vi "Write Pressure Alarm Level.vi"(8 "error in (no error)":errorcluster, 10 "Pressure Alarm Level":dbl format="%^_3g", 11 "Pressure Monitor in":refnum<class "Pressure Monitor.lvclass">) -> (0 "error out":errorcluster, 3 "Pressure Monitor out":refnum<class "Pressure Monitor.lvclass">)   [LabVIEW 2022 SP3, in "Pressure Monitor.lvclass"]
uses:
  Pressure Monitor.lvclass
  Pressure Monitor.lvclass/Pressure Monitor.ctl
  Pressure Settings.ctl
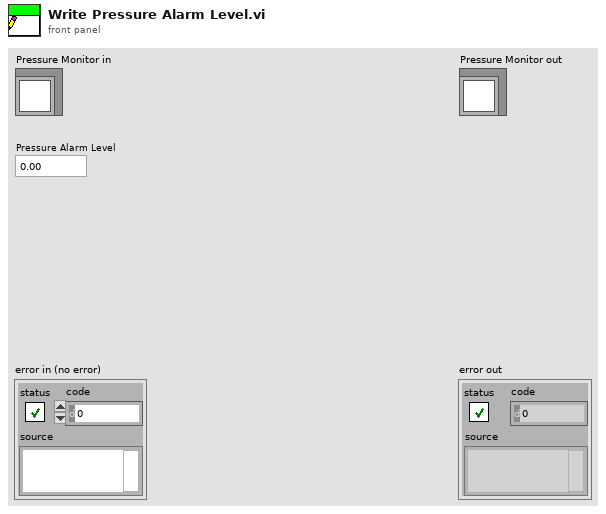
[diagram p1: front panel]
types:
  T1 = typedef "Pressure Monitor.lvclass/Pressure Settings.ctl" = cluster{"Pressure Alarm Level":dbl}
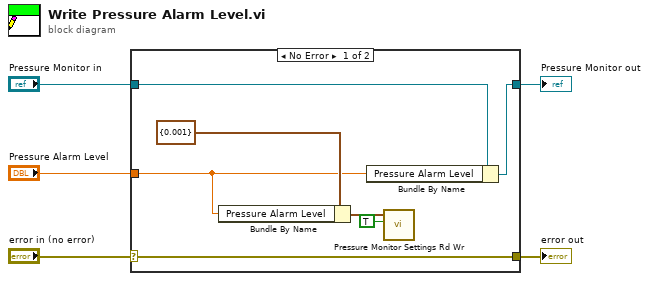
[diagram p0: block diagram]
diagram:
  n1 = case shown="No Error" "error in (no error)" {
    selector: "error in (no error)" -> [w12 w13]
    tunnel: [w12 w13] -> w4
    tunnel: [w10 w14] -> w2
    tunnel: "Pressure Monitor in" -> [w11 w14]
    tunnel: "Pressure Alarm Level" -> [w8 _]
    frame No Error {
      n2 = Bundle By Name(cluster=T1 {"Pressure Alarm Level"=0.001} ("Pressure Settings"), "Pressure Alarm Level"=w8) -> (w7:T1)
      n3 = Bundle By Name(cluster=w11, "Pressure Alarm Level"=w8) -> (w10:refnum<class "Pressure Monitor.lvclass">)
      n4 = call "Pressure Monitor Settings Rd Wr.vi"("Write? (F:Read)"=TRUE, "Pressure Settings"=w7) -> ()  [unwired: 8 in, 2 out]
    }
    frame Error {
    }
  }
  "error out" <- w4
  "Pressure Monitor out" <- w2
